vi "NI VeriStand - Set Calibration.vi"(8 "error in":errorcluster, 9 "Coefficients":dbl[](array[numeric]), 10 "Channel Name":string, 11 "Calibration In":T1) -> (0 "error out":errorcluster, 3 "Calibration Out":T1)   [LabVIEW 2020, in "NI_VS Calibration ExecutionAPI.lvlib"]
doc: "Applies a polynomial calibration to the specified channel, as defined by the <B>Coefficients</B> you specify."
uses:
  <vilib>/NI VeriStand/Execution/Calibration/NI_VS Calibration ExecutionAPI.lvlib
  <vilib>/NI VeriStand/Execution/Calibration/CalibrationAPI.ctl
  NationalInstruments.VeriStand.ClientAPI
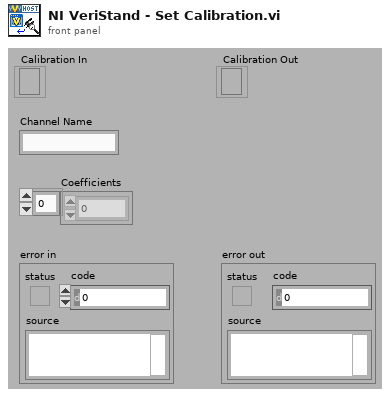
[diagram p1: front panel]
types:
  T1 = typedef "NI_VS Calibration ExecutionAPI.lvlib/CalibrationAPI.ctl" = refnum<k24>
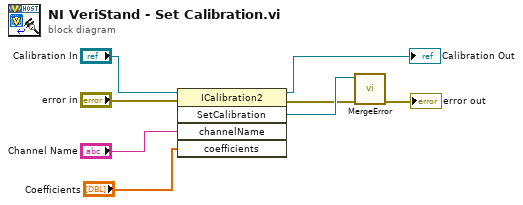
[diagram p0: block diagram]
diagram:
  n1 = invoke class="ICalibration2" method="SetCalibration"(reference="Calibration In", error in="error in", "channelName"="Channel Name", "coefficients"="Coefficients") -> (reference out=→"Calibration Out":T1, error out=w4:errorcluster, "SetCalibration"=w7:refnum<k24>)  [unwired: 1 in, 2 out]
  n2 = call <vilib>:"MergeError.vi"("error in (no error)"=w4, "Error"=w7) -> ("error out"=→"error out":errorcluster)  [unwired: 9 out]
